vi "GetColoredPen.vi"(0 "reference in":refnum<class "LcPictureBox.lvclass">, 1 "Alpha(100%)":dbl, 2 "Color(Black)":u32, 3 "Pen(Width=1, Solid)":T1, 5 "Error In":errorcluster) -> (14 "reference out":refnum<class "LcPictureBox.lvclass">, 15 "PenRef":refnum<k24>, 19 "Error Out":errorcluster)   [LabVIEW 2020, in "LcPictureBox.lvclass"]
uses:
  LcPictureBox.lvclass
  System.Drawing
  Pen.ctl
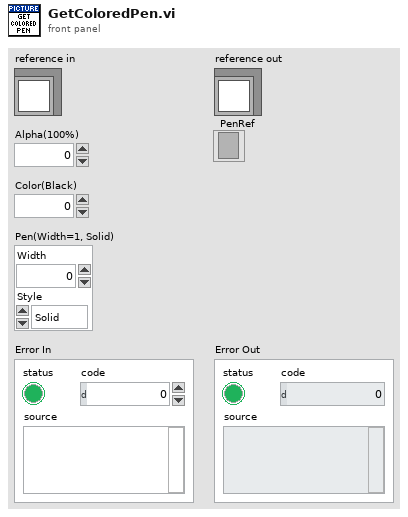
[diagram p1: front panel]
types:
  T1 = typedef "LcPictureBox.lvclass/Pen.ctl" = cluster{"Width":u16, "Style":enum32{"Solid", "Dash", "Dot", "DashDot", "DashDotDot"}}
  T2 = cluster{"Alpha(100%)":dbl, "Color(Black)":u32, "Pen(Width=1, Solid)":T1}
  T3 = typedef "LcPictureBox.lvclass/ObjectAttributes.ctl" = cluster{"PictureBox":refnum<k24>, "ImageSize":cluster{"Width":i32, "Height":i32}, "PenMemory":map{cluster{"Alpha(100%)":dbl, "Color(Black)":u32, "Pen(Width=1, Solid)":T1}, refnum<k24>}, "GraphicsRef":refnum<k24>, "BrushMemory":map{cluster{"Alpha(100%)":dbl, "Color(Black)":u32}, refnum<k24>}, "Images":refnum<k24>[], "ImageIndex":i32, "BgColor(None)":u32, "LoadedImages":map{string, cluster{"ImageOut":refnum<k24>, "ImageSize":cluster{"Width":i32, "Height":i32}}}, "ColorsMemory":map{cluster{"Alpha(100%)":dbl, "Color(Black)":u32}, refnum<k24>}, "CacheSize":i32, "PictureBoxActiveXReference":refnum<vi>, "Scale":sgl, "Offset":cluster{"x":sgl, "y":sgl}, "zoom_center":cluster{"X":i32, "Y":i32}, "ImagesCreated":refnum<k24>[]}
  T4 = map{cluster{"Alpha(100%)":dbl, "Color(Black)":u32}, refnum<k24>}
  T5 = map{cluster{"Alpha(100%)":dbl, "Color(Black)":u32, "Pen(Width=1, Solid)":T1}, refnum<k24>}
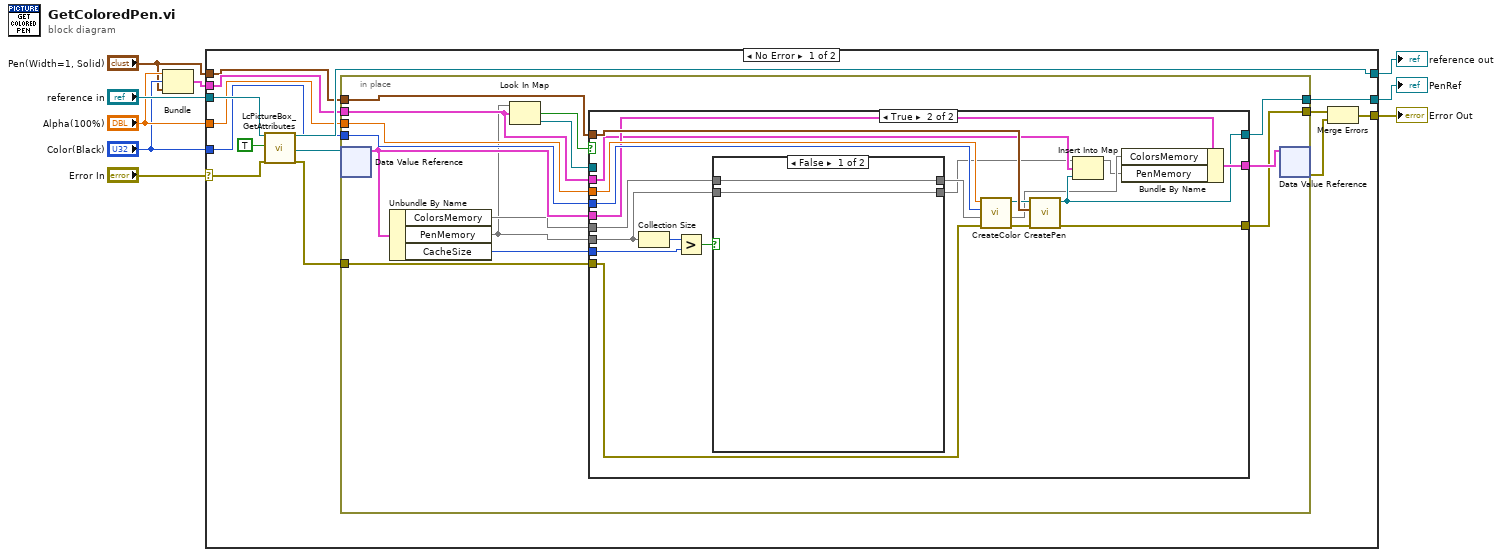
[diagram p0: block diagram]
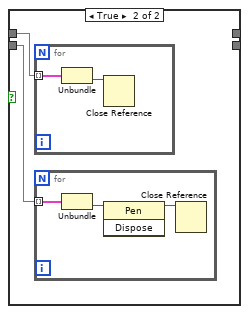
[diagram p3: hidden frame]
diagram:
  n1 = Bundle("Alpha(100%)"="Alpha(100%)", "Color(Black)"="Color(Black)", "Pen(Width=1, Solid)"="Pen(Width=1, Solid)") -> (w5:T2)  [unwired: 1 in]
  n2 = case shown="No Error" "Error In" {
    selector: "Error In" -> [w22 w71]
    tunnel: [w19 w71] -> w8
    tunnel: [w20 w70] -> w6
    tunnel: "reference in" -> [w23 w70]
    tunnel: w5 -> [w16 _]
    tunnel: [w15 _] -> w4
    tunnel: "Alpha(100%)" -> [w14 _]
    tunnel: "Color(Black)" -> [w13 _]
    tunnel: "Pen(Width=1, Solid)" -> [w12 _]
    frame No Error {
      n3 = call "LcPictureBox_GetAttributes.vi"("reference in"=w23, "OnlyGetDvrReference(False)"=TRUE, "error in (no error)"=w22) -> ("reference out"=w20:refnum<class "LcPictureBox.lvclass">, "DataRef"=w18:refnum<data-value>, "error out"=w11:errorcluster)  [unwired: 13 in, 1 out]
      n4 = in-place {
        in-place-border: w16 -> [w27]
        in-place-border: [w33] -> w15
        in-place-border: w14 -> [w32]
        in-place-border: w13 -> [w31]
        in-place-border: w11 -> [w30]
        in-place-border: w12 -> [w29]
        in-place-border: [w28] -> w10
        n5 = in-place-dvr #1(w18) -> (w36:T3)  [unwired: 1 out]
        n6 = Unbundle By Name(w36) -> ("ColorsMemory"=w26:T4, "PenMemory"=w25:T5, "CacheSize"=w24:i32)
        n7 = Look In Map(map=w25, key=w27) -> (key not found?=w35:bool, value=w34:refnum<k24>)  [unwired: 1 in]
        n8 = case shown="True" w35 {
          tunnel: [w38 w60] -> w37
          tunnel: w36 -> [w38 w54]
          tunnel: w34 -> [w40 _]
          tunnel: [w40 w52] -> w33
          tunnel: w32 -> [_ w59]
          tunnel: w31 -> [_ w58]
          tunnel: w30 -> [w39 w57]
          tunnel: w29 -> [_ w55]
          tunnel: [w39 w50] -> w28
          tunnel: w25 -> [_ w44]
          tunnel: w27 -> [_ w53]
          tunnel: w26 -> [_ w46]
          tunnel: w24 -> [_ w48]
          frame False {
          }
          frame True {
            n9 = Collection Size(1:w44) -> (0:w49:i32)
            n10 = Greater?(x=w49, y=w48) -> (0:w47:bool)
            n11 = case shown="False" w47 {
              tunnel: w46 -> [w62 w63]
              tunnel: w44 -> [w61 w64]
              tunnel: [w62 _] -> w45
              tunnel: [w61 _] -> w43
              frame False {
              }
              frame True {
                n12 = for {
                  tunnel: w63 -> [w66] mode=indexing
                  n13 = Unbundle(w66) -> ("ColorRef"=w65:refnum<k24>)  [unwired: 1 out]
                  n14 = Close Reference(reference=w65) -> ()  [unwired: 1 in, 1 out]
                }
                n15 = for {
                  tunnel: w64 -> [w69] mode=indexing
                  n16 = Unbundle(w69) -> ("PenRef"=w68:refnum<k24>)  [unwired: 1 out]
                  n17 = invoke class="Pen" method="Dispose"(reference=w68) -> (reference out=w67:refnum<k24>)  [unwired: 2 in, 2 out]
                  n18 = Close Reference(reference=w67) -> ()  [unwired: 1 in, 1 out]
                }
              }
            }
            n19 = call "CreateColor.vi"("error in (no error)"=w57, "ColorsIn"=w45, "Color(Black)"=w58, "Alpha(100%)"=w59) -> ("error out"=w56:errorcluster, "ColorsOut"=w42:T4, "ColorRef"=w51:refnum<k24>)  [unwired: 5 in]
            n20 = call "CreatePen.vi"("error in (no error)"=w56, "Pen(Width=1, Solid)"=w55, "ColorRef"=w51) -> ("error out"=w50:errorcluster, "PenRef"=w52:refnum<k24>)  [unwired: 7 in]
            n21 = Insert Into Map(map in=w43, key=w53, value=w52) -> (map out=w41:T5)  [unwired: 2 out]
            n22 = Bundle By Name(cluster=w54, "ColorsMemory"=w42, "PenMemory"=w41) -> (w60:T3)
          }
        }
        n23 = in-place-dvr #1(w37) -> (w21:errorcluster)  [unwired: 1 out]
      }
      n24 = Merge Errors(w10, w21) -> (w19:errorcluster)
    }
    frame Error {
    }
  }
  "Error Out" <- w8
  "reference out" <- w6
  "PenRef" <- w4
